vi "Read ROI.vi"(8 "error in (no error)":errorcluster, 11 "Camera Data in":refnum<class "Camera Data.lvclass">) -> (0 "error out":errorcluster, 2 "ROI":T1, 3 "Camera Data out":refnum<class "Camera Data.lvclass">)   [LabVIEW 2022 SP3, in "Camera Data.lvclass"]
uses:
  Camera Data.lvclass
  Camera Data.lvclass/Camera Data.ctl
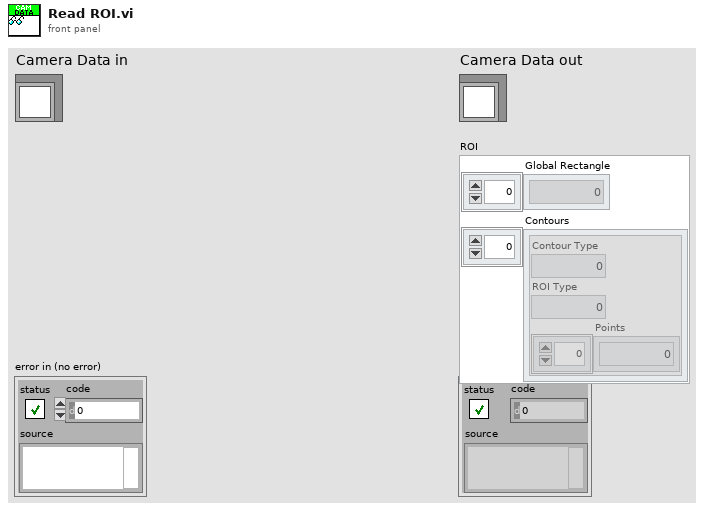
[diagram p1: front panel]
types:
  T1 = cluster{"Global Rectangle":i32[], "Contours":cluster{"Contour Type":u32, "ROI Type":u32, "Points":i32[]}[]}
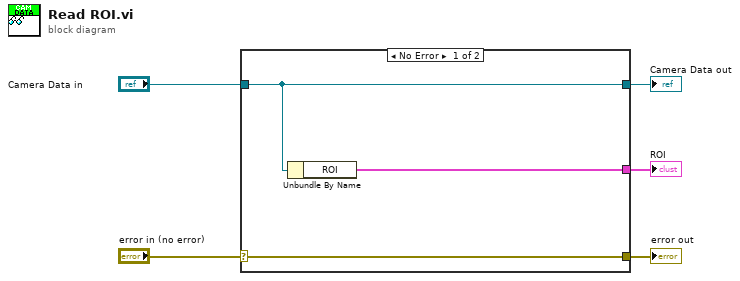
[diagram p0: block diagram]
diagram:
  n1 = case shown="No Error" "error in (no error)" {
    selector: "error in (no error)" -> [w8 w9]
    tunnel: [w8 w9] -> w4
    tunnel: [w7 w10] -> w2
    tunnel: "Camera Data in" -> [w7 w10]
    tunnel: [w6 _] -> w1
    frame No Error {
      n2 = Unbundle By Name(w7) -> ("ROI"=w6:T1)
    }
    frame Error {
    }
  }
  "error out" <- w4
  "Camera Data out" <- w2
  "ROI" <- w1
